vi "BITMAPINFOHEADER.vi"(11 "Image Dimensions":i32[](array[numeric])) -> (3 "BITMAPFILEHEADER":u8[](array[numeric]))   [LabVIEW 2012]
panel:
  out "size(s)":i32
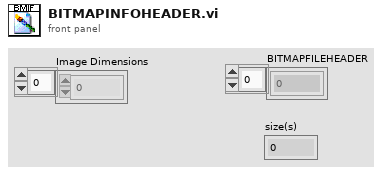
[diagram p1: front panel]
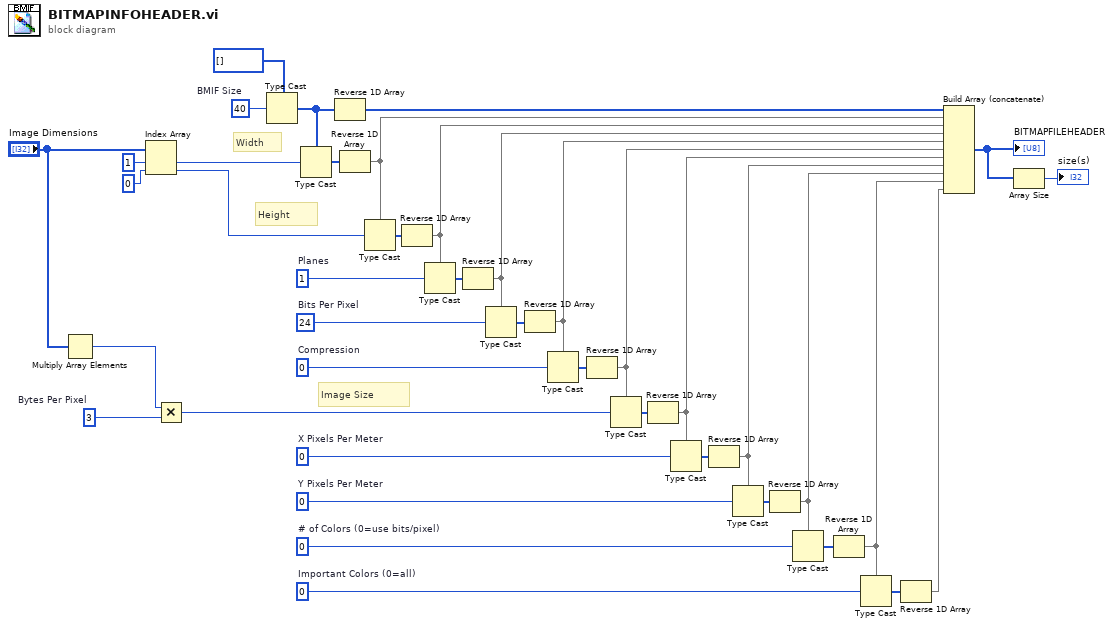
[diagram p0: block diagram]
diagram:
  w26 = 3  # Bytes Per Pixel
  w29 = 0  # Important Colors (0=all)
  w30 = 0  # # of Colors (0=use bits/pixel)
  w33 = 0  # Y Pixels Per Meter
  w34 = 0  # X Pixels Per Meter
  w35 = 0  # Compression
  w36 = i16 24  # Bits Per Pixel
  w37 = i16 1  # Planes
  w38 = 40  # BMIF Size
  # "Image Size"
  # "Height"
  # "Width"
  n1 = Multiply Array Elements(1:"Image Dimensions") -> (0:w2:i32)
  n2 = Index Array(array="Image Dimensions", index #1=1 ("index"), index #2=0 ("index")) -> (element #1=w27:i32, element #2=w28:i32)
  n3 = Multiply(x=w2, y=w26) -> (x*y=w1:i32)
  n4 = Type Cast(type=u8[] [], x=w38) -> (*(type *) &x=w7:u8[])
  n5 = Type Cast(type=w7, x=w27) -> (*(type *) &x=w25:u8[])
  n6 = Reverse 1D Array(array=w7) -> (reversed array=w6:u8[])
  n7 = Reverse 1D Array(array=w25) -> (reversed array=w24:u8[])
  n8 = Type Cast(type=w24, x=w28) -> (*(type *) &x=w23:u8[])
  n9 = Reverse 1D Array(array=w23) -> (reversed array=w22:u8[])
  n10 = Type Cast(type=w22, x=w37) -> (*(type *) &x=w21:u8[])
  n11 = Reverse 1D Array(array=w21) -> (reversed array=w20:u8[])
  n12 = Type Cast(type=w20, x=w36) -> (*(type *) &x=w19:u8[])
  n13 = Reverse 1D Array(array=w19) -> (reversed array=w18:u8[])
  n14 = Type Cast(type=w18, x=w35) -> (*(type *) &x=w17:u8[])
  n15 = Reverse 1D Array(array=w17) -> (reversed array=w16:u8[])
  n16 = Type Cast(type=w16, x=w1) -> (*(type *) &x=w15:u8[])
  n17 = Reverse 1D Array(array=w15) -> (reversed array=w14:u8[])
  n18 = Type Cast(type=w14, x=w34) -> (*(type *) &x=w13:u8[])
  n19 = Reverse 1D Array(array=w13) -> (reversed array=w12:u8[])
  n20 = Type Cast(type=w12, x=w33) -> (*(type *) &x=w11:u8[])
  n21 = Reverse 1D Array(array=w11) -> (reversed array=w10:u8[])
  n22 = Type Cast(type=w10, x=w30) -> (*(type *) &x=w9:u8[])
  n23 = Reverse 1D Array(array=w9) -> (reversed array=w8:u8[])
  n24 = Type Cast(type=w8, x=w29) -> (*(type *) &x=w5:u8[])
  n25 = Reverse 1D Array(array=w5) -> (reversed array=w4:u8[])
  n26 = Build Array (concatenate)(w6, w24, w22, w20, w18, w16, w14, w12, w10, w8, w4) -> (w32:u8[])
  "BITMAPFILEHEADER" <- w32
  n27 = Array Size(array=w32) -> (size(s)=→"size(s)":i32)
